vi "TellSelf.vi"(6 "Error":errorcluster, 10 "PayloadCluster":T1 {"MetadataCluster"."AbsoluteTime" format="%<%x %.3X>T"}, 11 "Actor":refnum<class "Actor.lvclass">) -> (3 "Actor":refnum<class "Actor.lvclass">, 4 "Error":errorcluster)   [LabVIEW 2020, in "_Template.lvlib" / "{{Message}}.lvlib"]
uses:
  {{Message}}.lvlib
  Message/Message.lvclass
  C:/jettl-harness/repos/jettl/src/jettl Tools/_Template/{{Message}}/Message/Message.lvclass
  C:/jettl-harness/repos/jettl/src/jettl/jettl/Message/Message.lvclass
  jettl/jettl/jettl.lvlib
  jettl/jettl/Actor/Actor.lvclass
  jettl/jettl/LifecycleEnum.ctl
  jettl/jettl/MetadataCluster.ctl
  PayloadCluster.ctl
  jettl/jettl/TellOriginEnum.ctl
  jettl/jettl/CustomMetadata/CustomMetadata.lvclass
panel:
  # "This front panel should not be manipulated."
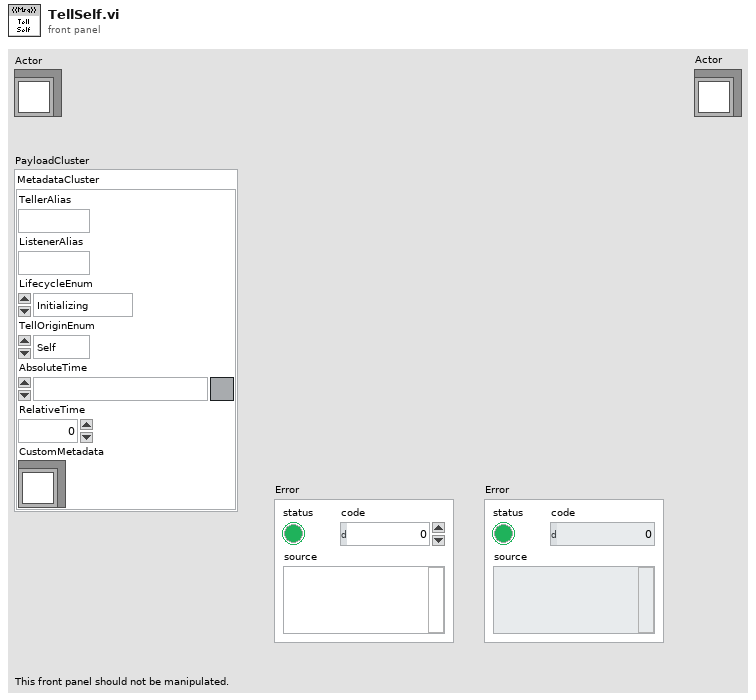
[diagram p1: front panel]
types:
  T1 = typedef "_Template.lvlib/{{Message}}.lvlib/PayloadCluster.ctl" = cluster{"MetadataCluster":T2}
  T2 = typedef "jettl.lvlib/MetadataCluster.ctl" = cluster{"TellerAlias":string, "ListenerAlias":string, "LifecycleEnum":T3, "TellOriginEnum":T4, "AbsoluteTime":timestamp, "RelativeTime":dbl, "CustomMetadata":refnum<class "CustomMetadata.lvclass">}
  T3 = typedef "jettl.lvlib/LifecycleEnum.ctl" = enum16{"Initializing", "SettingUp", "Starting", "Running", "Stopping", "TearingDown", "Terminated", "Abort"}
  T4 = typedef "jettl.lvlib/TellOriginEnum.ctl" = enum16{"Self", "Mediator", "Component"}
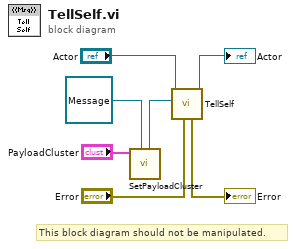
[diagram p0: block diagram]
diagram:
  # "This block diagram should not be manipulated."
  n1 = call "SetPayloadCluster.vi"("Message"=refnum<class "Message.lvclass"> refnum ("_Template.lvlib:MessageTemplate.lvlib:{{Name}}.lvlib:ConcreteMessage.lvclass"), "PayloadCluster"="PayloadCluster") -> ("Message"=w4:refnum<class "Message.lvclass">)  [unwired: 9 in]
  n2 = call "TellSelf.vi"("Error"="Error", "Message"=w4, "Actor"="Actor") -> ("Actor"=→"Actor":refnum<class "Actor.lvclass">, "Error"=→"Error":errorcluster)  [unwired: 7 in]
